vi "Label Targets2.vi"(7 "Annotate":bool=TRUE, 10 "Results":T2 {"Score" format="%#_3g"; "Pixels"."Rectangle"."Numeric 5" format="%#_3g"; "Pixels"."Rectangle"."Numeric 3" format="%#_3g"; "Pixels"."Rectangle"."Numeric 2" format="%#_3g"; "Pixels"."Rectangle"."Numeric" format="%#_3g"; "Normalized"."Rectangle"."Numeric 5" format="%#_2g"; "Normalized"."Rectangle"."Numeric 3" format="%#_2g"; "Normalized"."Rectangle"."Numeric 2" format="%#_2g"; "Normalized"."Rectangle"."Numeric" format="%#_2g"; "Normalized"."Center"."?" format="%#_3g"; "Normalized"."Center"."?" format="%#_3g"; "Distance (ft)" format="%#_3g"}, 11 "Image in":T1) -> (3 "Image out":T1)   [LabVIEW 2018]
doc: "Draw text values near or on the particle and draws a square around the target stripes.."
uses:
  <vilib>/vision/Image Controls.llb/IMAQ Image.ctl
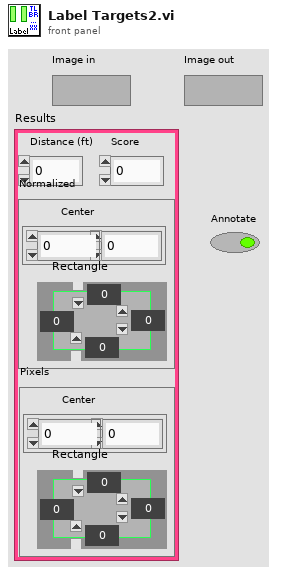
[diagram p1: front panel]
types:
  T1 = typedef "IMAQ Image.ctl" = refnum<image>
  T2 = cluster{"Distance (ft)":dbl, "Score":dbl, "Normalized":cluster{"Center":cluster{dbl, dbl}, "Rectangle":cluster{"Numeric":dbl, "Numeric 2":dbl, "Numeric 3":dbl, "Numeric 5":dbl}}, "Pixels":cluster{"Center":cluster{dbl, dbl}, "Rectangle":cluster{"Numeric":dbl, "Numeric 2":dbl, "Numeric 3":dbl, "Numeric 5":dbl}}}
  T3 = cluster{"Desired Font (Application)":enum16{"User-specified Font", "Application Font", "System Font", "Dialog Font"}, "[User-specified Font]":cluster{"Font Name":string, "Size":i16, "Strikeout?":bool, "Italic?":bool, "Underline?":bool, "Outline?":bool, "Shadow?":bool, "Bold?":bool, "Rotation Angle":dbl}, "Horizontal Alignment":i16, "Vertical Alignment":i16}
  T4 = cluster{"Center":cluster{dbl, dbl}, "Rectangle":cluster{"Numeric":dbl, "Numeric 2":dbl, "Numeric 3":dbl, "Numeric 5":dbl}}
  T5 = cluster{"Numeric":dbl, "Numeric 2":dbl, "Numeric 3":dbl, "Numeric 5":dbl}
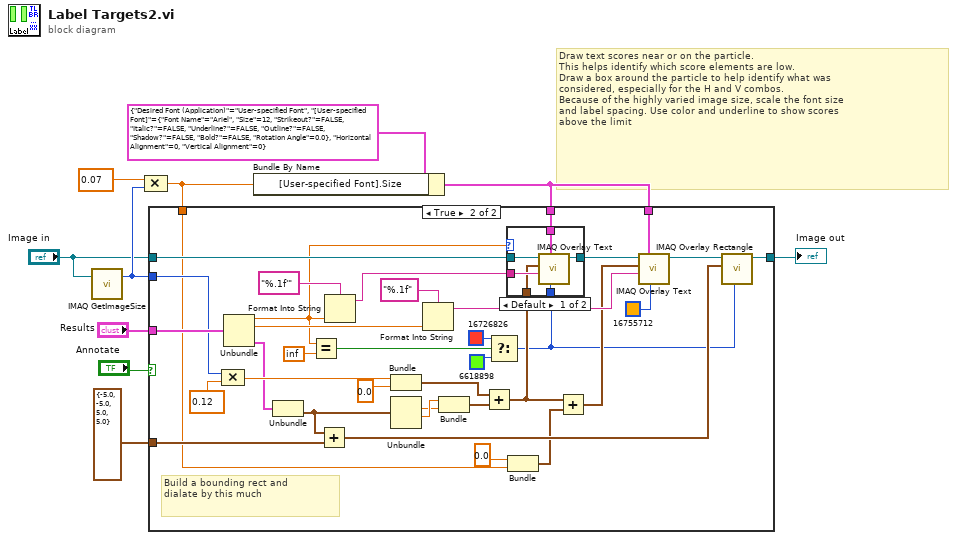
[diagram p0: block diagram]
diagram:
  # "Draw text scores near or on the particle.\nThis helps identify which score elements are low.\nDraw a box around the particle to help identify what was\nconsidered, especially for the H and V combos.\nBecause of the highly varied image size, scale the font size\nand label spacing. Use color and underline to show scores\nabove the limit"
  n1 = call "IMAQ GetImageSize"("Image"="Image in") -> ("Y Resolution"=w6:i32)  [unwired: 3 in, 2 out]
  n2 = Compound Arithmetic op=MULTIPLY(0.07, w6) -> (w2:dbl)
  n3 = Bundle By Name(cluster=T3 {"Desired Font (Application)"=enum."User-specified Font", "[User-specified Font]"={"Font Name"="Ariel", "Size"=12, "Strikeout?"=FALSE, "Italic?"=FALSE, "Underline?"=FALSE, "Outline?"=FALSE, "Shadow?"=FALSE, "Bold?"=FALSE, "Rotation Angle"=0.0}, "Horizontal Alignment"=0, "Vertical Alignment"=0} ("Font, Size & Style"), "[User-specified Font].Size"=w2) -> (w3:T3)
  n4 = case shown="True" "Annotate" {
    tunnel: [w11 w12] -> w10
    tunnel: "Results" -> [_ w47]
    tunnel: "Image in" -> [w11 w46]
    tunnel: w3 -> [_ w35]
    tunnel: w6 -> [_ w45]
    tunnel: cluster{dbl, dbl, dbl, dbl} {-5.0, -5.0, 5.0, 5.0} ("output cluster") -> [_ w34]
    tunnel: w3 -> [_ w29]
    tunnel: w2 -> [_ w20]
    frame False {
    }
    frame True {
      # "Build a bounding rect and\ndialate by this much"
      n5 = Compound Arithmetic op=MULTIPLY(w45, 0.12) -> (w38:dbl)
      n6 = Unbundle(w47) -> ("Distance (ft)"=w13:dbl, "Score"=w27:dbl, "Pixels"=w32:T4)  [unwired: 1 out]
      n7 = Unbundle(w32) -> ("Rectangle"=w33:T5)  [unwired: 1 out]
      n8 = Equal?(x=w13, y=inf) -> (x = y?=w16:bool)
      n9 = Add(x=w33, y=w34) -> (x+y=w41:cluster{dbl, dbl, dbl, dbl})
      n10 = Format Into String(format string="%.1f'", w13) -> (resulting string=w36:string)  [unwired: 2 in, 1 out]
      n11 = Bundle(w38, 0.0) -> (w40:cluster{dbl, dbl})  [unwired: 1 in]
      n12 = Unbundle(w33) -> ("Numeric 2"=w43:dbl, "Numeric 3"=w44:dbl)  [unwired: 2 out]
      n13 = Format Into String(format string="%.1f", w27) -> (resulting string=w25:string)  [unwired: 2 in, 1 out]
      n14 = Bundle("Numeric 3"=w44, "Numeric 2"=w43) -> (w42:cluster{"Numeric 3":dbl, "Numeric 2":dbl})  [unwired: 1 in]
      n15 = Add(x=w40, y=w42) -> (x+y=w24:cluster{dbl, dbl})
      n16 = Select(t=u32 16726826 ("Color"), s=w16, f=u32 6618898 ("Color")) -> (s? t:f=w14:u32)
      n17 = case shown="Default" w13 {
        tunnel: w46 -> [w53 w54]
        tunnel: w36 -> [w52 _]
        tunnel: w35 -> [w51 _]
        tunnel: [w50 w54] -> w31
        tunnel: w24 -> [w49 _]
        tunnel: w14 -> [w48 _]
        frame Default {
          n18 = call "IMAQ Overlay Text"("Text Color (black)"=w48, "Font, Size & Style"=w51, "String"=w52, "Origin"=w49, "Image"=w53) -> ("Image Out"=w50:T1)  [unwired: 5 in, 1 out]
        }
        frame 0 {
        }
      }
      n19 = Bundle(0.0, w20) -> (w23:cluster{dbl, dbl})  [unwired: 1 in]
      n20 = Add(x=w24, y=w23) -> (x+y=w21:cluster{dbl, dbl})
      n21 = call "IMAQ Overlay Text"("Text Color (black)"=u32 16755712 ("Color"), "Font, Size & Style"=w29, "String"=w25, "Origin"=w21, "Image"=w31) -> ("Image Out"=w30:T1)  [unwired: 5 in, 1 out]
      n22 = call "IMAQ Overlay Rectangle"("Color"=w14, "Rectangle"=w41, "Image"=w30) -> ("Image Out"=w12:T1)  [unwired: 7 in, 1 out]
    }
  }
  "Image out" <- w10
